vi "ConvertChannelsArrayToString.vi"(8 "error in (no error)":errorcluster, 10 "Channels in":T1) -> (0 "error out":errorcluster, 1 "String array":string[](array[string]), 2 "String":string)   [LabVIEW 2016, in "pickering.lvclass"]
uses:
  pickering.lvclass
  Typedefs/Channels-Array.ctl
  Typedefs/Channel-Cluster.ctl
  Typedefs/ChannelX-ComboBox.ctl
  Typedefs/ChannelY-ComboBox.ctl
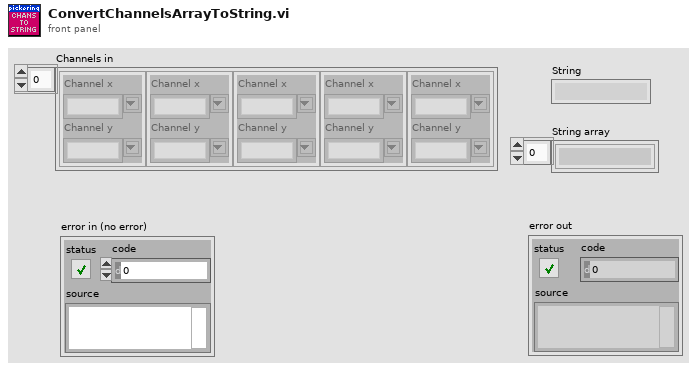
[diagram p1: front panel]
types:
  T1 = typedef "pickering.lvclass/Channels-Array.ctl" = T2[]
  T2 = typedef "pickering.lvclass/Channel-Cluster.ctl" = cluster{"Channel x":T3, "Channel y":T4}
  T3 = typedef "pickering.lvclass/ChannelX-ComboBox.ctl" = string
  T4 = typedef "pickering.lvclass/ChannelY-ComboBox.ctl" = string
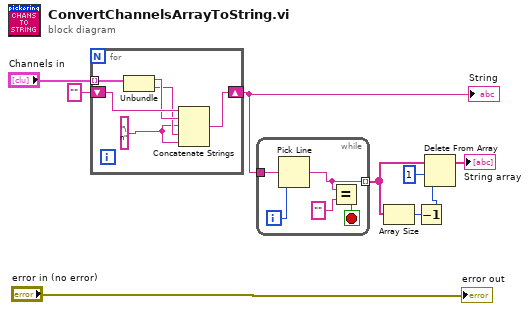
[diagram p0: block diagram]
diagram:
  n1 = for {
    tunnel: "Channels in" -> [w15] mode=indexing
    shift-right: [w14] -> w2
    shift-left: "" -> [w13]
    w10 = "\n"
    n2 = Unbundle(w15) -> ("Channel x"=w12:T3, "Channel y"=w11:T4)
    n3 = Concatenate Strings(w13, w12, w10, w11, w10) -> (w14:string)
  }
  "String" <- w2
  n4 = while {
    tunnel: w2 -> [w20]
    tunnel: [w18] -> w6 mode=indexing
    i -> [w19]
    stop <- w16 stop-if-true
    n5 = Pick Line(multi-line string=w20, line index=w19) -> (output string=w18:string)  [unwired: 1 in]
    n6 = Equal?(x=w18, y="" ("output string")) -> (x = y?=w16:bool)
  }
  n7 = Array Size(array=w6) -> (size(s)=w3:i32)
  n8 = Decrement(x=w3) -> (x-1=w4:i32)
  n9 = Delete From Array(array=w6, length=1, index=w4) -> (array with subset deleted=→"String array":string[])  [unwired: 1 out]
  "error out" <- "error in (no error)"
